vi "send_array.vi"() -> ()   [LabVIEW 2013]
panel:
  in  "data":u16
  in  "elemszam":u16
  out "error out":errorcluster
  out "VISA resource name out":refnum<visa-resource-name>
  in  "VISA resource name 3":refnum<visa-resource-name>
  in  "error in (no error) 3":errorcluster
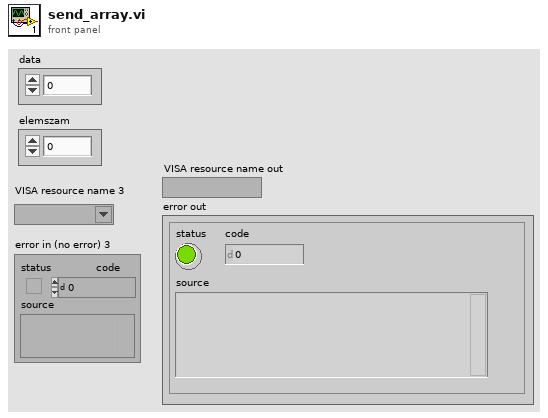
[diagram p1: front panel]
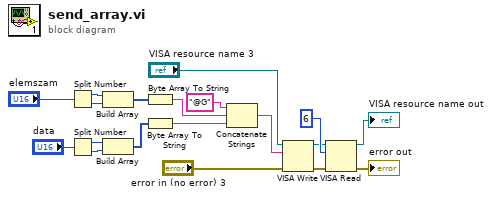
[diagram p0: block diagram]
diagram:
  n1 = Split Number(x="elemszam") -> (hi(x)=w9:u8, lo(x)=w8:u8)
  n2 = Split Number(x="data") -> (hi(x)=w4:u8, lo(x)=w3:u8)
  n3 = Build Array(w9, w8) -> (w7:u8[])
  n4 = Build Array(w4, w3) -> (w2:u8[])
  n5 = Byte Array To String(unsigned byte array=w7) -> (string=w6:string)
  n6 = Byte Array To String(unsigned byte array=w2) -> (string=w1:string)
  n7 = Concatenate Strings("@G" ("write buffer"), w6, w1) -> (w16:string)
  n8 = VISA Write(VISA resource name="VISA resource name 3", write buffer=w16, error in (no error)="error in (no error) 3") -> (VISA resource name out=w14:refnum<visa-resource-name>, error out=w13:errorcluster)  [unwired: 1 out]
  n9 = VISA Read(VISA resource name=w14, byte count=u32 6, error in (no error)=w13) -> (VISA resource name out=→"VISA resource name out":refnum<visa-resource-name>, error out=→"error out":errorcluster)  [unwired: 2 out]
